vi "Stufen testen.vi"(4 "GD LNI old":bool, 7 "Komponentenauswahl":T5 {"Konzentration" format="%#.6f"}, 8 "error in (no error)":errorcluster caption="Fehler (Eingang, kein Fehler)", 9 "Index Cluster":T4 {"Verdünnungsgas" items=["N2", "O2"]; "Anzahl Stufen" format="%#_5g"}) -> (0 "error out":errorcluster caption="Fehler (Ausgang)", 2 "GD DF":T1)   [LabVIEW 2020, in "Linearisierung v2.lvlib" / "Gasteiler.lvlib"]
uses:
  Gasteiler.lvlib
  KomponentenArray.ctl
  Visualisierungs Elemente/Auswahlfeld.ctl
  Visualisierungs Elemente/Zahlen-Eingabefeld.ctl
  Visualisierungs Elemente/Checkbox(boolsch).ctl
  Aktionen FGV Gasteiler Daten.ctl
  SpanEinstellungen/Aktion FGV GD Errors sammeln.ctl
  SpanEinstellungen/GD Info Cluster.ctl
  LIN ErrorCluster.ctl
  Aktion FGV Gasteilerliste laden.ctl
  AK-Komm Gasteiler/Aktionen AK Komm.ctl
  AK-Komm Gasteiler/Alter Gasteiler/Aktionen AK Komm_ALT.ctl
  Seiten/System Einstellungen V2/Traegergas.ctl
  Horiba/Aktion Befehl.ctl
  Gasteiler Fehler.ctl
  Aktion Lin Daten aufarbeiten.ctl
  Linearisierung v2.lvlib
  Seiten/System Einstellungen V2/System Einstellungen V2.lvlib
  SpanEinstellungen/SpanEinstellungen.lvlib
  AK-Komm Gasteiler/AK Komm Gasteiler.lvlib
  AK-Komm Gasteiler/Alter Gasteiler/Alter Gasteiler.lvlib
  Horiba/Horiba GDC.lvlib
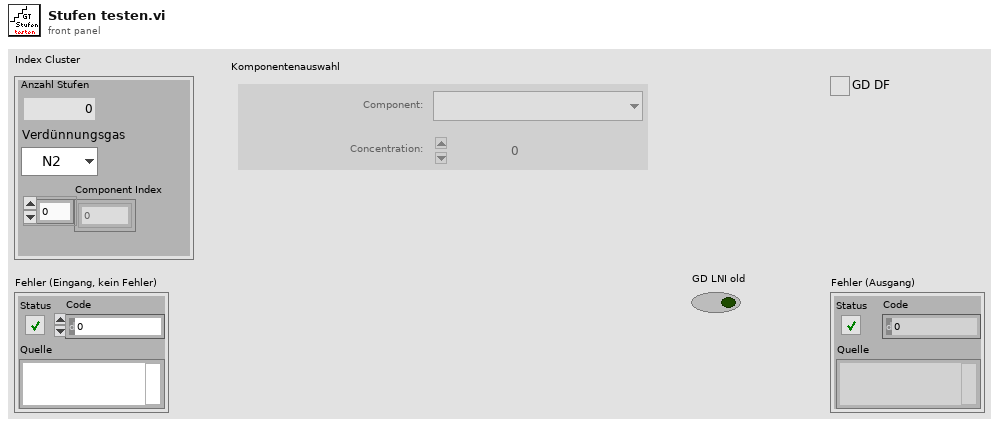
[diagram p1: front panel]
types:
  T1 = typedef "Checkbox(boolsch).ctl" = bool
  T2 = typedef "Zahlen-Eingabefeld.ctl" = sgl
  T3 = typedef "Linearisierung v2.lvlib/Gasteiler.lvlib/Prüfgas in.ctl" = u16
  T4 = cluster{"Anzahl Stufen":T2, "Verdünnungsgas":T3, "Component Index":i32[]}
  T5 = typedef "Linearisierung v2.lvlib/KomponentenArray.ctl" = cluster{"Komponente:":T6, "Konzentration":dbl}[]
  T6 = typedef "Auswahlfeld.ctl" = u16
  T7 = typedef "Linearisierung v2.lvlib/SpanEinstellungen.lvlib/GD Info Cluster.ctl" = cluster{"Wobei":string, "Status":string, "Errors":T8, "Empfangsdaten":string[], "Zeitstempel":string}
  T8 = typedef "Linearisierung v2.lvlib/LIN ErrorCluster.ctl" = cluster{"Störung Kommunikation":bool, "Pressure carrier gas":bool, "Pressure diluted gas":bool, "Outlet Pressure":bool, "SNOX before SAIR":bool, "Störung Gasteiler":bool}
  T9 = typedef "Linearisierung v2.lvlib/SpanEinstellungen.lvlib/Aktion FGV GD Errors sammeln.ctl" = enum16{"lesen", "init", "GD Infos sammeln", "Kalibrierinfos sammeln", "Test Data", "GD Infos selektiv sammeln"}
  T10 = typedef "Linearisierung v2.lvlib/Gasteiler.lvlib/Aktionen FGV Gasteiler Daten.ctl" = enum16{"lesen", "Gasteiler Daten", "Seriellen Param.", "MB-Endwert", "laden", "speichern", "Anforderung", "TCP", "Aufzeichnung Start"}
  T11 = typedef "Linearisierung v2.lvlib/Aktion Lin Daten aufarbeiten.ctl" = enum16{"lesen", "Protkolldaten", "speichern", "laden", "EPA auswerten", "Tabelle schreiben", "Lin auswerten", "Tab init", "Stufentabelle", "EPA aktiviert", "Nachbehandlung laden", "Tabelle löschen", "Istwerte löschen", "Zeile löschen", "Zeile einfügen", "LIN aktiviert", "LIN/EPA aktiv laden", "EGAK Tab", "LIN übernehmen", "Tab init ohne Stufen"}
  T12 = typedef "Linearisierung v2.lvlib/Lin-Polynom Daten.ctl" = cluster{"Messgerät":string, "Kalibrator (Gasteiler)":string, "Bearbeiter/in":string, "Komponente":string, "Zeitstempel":timestamp, "F_max gefordert (%)":sgl, "F_max in %":sgl, "F_max in ppm":sgl, "Vorschlag Ordnung":i32, "Polynom OK":bool, "Polynomkoeff.":dbl[], "Prüfgas Konzentration":dbl, "Pfad EPA":string, "Pfad_LIN":string, "Gasnummer:":u8, "Komponentenauswahl":T5, "Verdünnungsgas":T3, "Zeitdauer Stufe":T2, "Anzahl Stufen":T2, "F_max in % EPA":sgl, "F_max in ppm EPA":sgl, "F_max in % LIN":sgl, "F_max in ppm LIN":sgl, "Punkte umkehren":bool, "EPA Optionsfeld":T13, "Autolin Hovacal":T14, "Spanfactors":sgl[], "Kalibrierauswahl":T15, "Conditions:":T16, "Gasflaschen Nr.:":string, "Bottle Accuracy":dbl, "Konfig Gasflasche":T17, "Gasflasche":T18, "HovaCAL Flow AutoLin":T19, "MFC Output":T20, "Gas Ablaufdatum":timestamp, "Lin Modus":T21, "zusätzliche Zeitdauer Erster Punkt":sgl, "Offsets":sgl[]}
  T13 = typedef "Linearisierung v2.lvlib/EPA Optionsfeld.ctl" = enum32{"Istwert", "Rohwert", "Linearisierter Wert"}
  T14 = typedef "Linearisierung v2.lvlib/Gasteiler.lvlib/HovaCal.lvlib/AutoLin Hovacal.ctl" = enum32{"Keine Auswahl", "Optionsauswahl 1", "Optionsauswahl 2"}
  T15 = typedef "Linearisierung v2.lvlib/Kalibrieroption.ctl" = u16
  T16 = typedef "Linearisierung v2.lvlib/Linearity verification 1065-307.lvlib/Condition.ctl" = u16
  T17 = typedef "System Einstellungen V2.lvlib/Konfig Gasflasche.ctl" = bool
  T18 = typedef "System Einstellungen V2.lvlib/Gasflasche Auswahl.ctl" = u16
  T19 = typedef "Linearisierung v2.lvlib/Gasteiler.lvlib/HovaCAL_Interface.lvlib/Controls.lvlib/Flow Einstellung.ctl" = cluster{"HovaCAL Flow Input Cluster":dbl}
  T20 = typedef "Linearisierung v2.lvlib/Gasteiler.lvlib/HovaCAL_Interface.lvlib/Controls.lvlib/Pump state.ctl" = cluster{"Run":bool}
  T21 = typedef "Linearisierung v2.lvlib/Lin Modus.ctl" = u16
  T22 = typedef "Linearisierung v2.lvlib/Gasteiler.lvlib/Aktion FGV Gasteilerliste laden.ctl" = enum16{"lesen", "laden", "speichern", "Liste erstellen", "Formel ändern", "Gas vereinzeln"}
  T23 = typedef "Linearisierung v2.lvlib/Gasteiler.lvlib/Gasteiler Daten.ctl" = cluster{"Gasteiler":T24, "Gasteiler Stufen":T25, "Gasteiler Type":T26, "Konfig Gasteiler":T27, "Gasteiler Span Eingänge":u16}
  T24 = typedef "String - Eingabefeld.ctl" = string
  T25 = typedef "Linearisierung v2.lvlib/Gasteiler.lvlib/Gasteiler Stufen.ctl" = u16
  T26 = typedef "Linearisierung v2.lvlib/GasteilerType.ctl" = u16
  T27 = typedef "System Einstellungen V2.lvlib/Gasteiler Auswahl.ctl" = u16
  T28 = typedef "Linearisierung v2.lvlib/Gasteiler.lvlib/AK Komm Gasteiler.lvlib/Aktionen AK Komm.ctl" = enum16{"lesen", "initialisieren", "beenden", "Status", "SMAN", "SREM", "STBY", "ASTF", "ASTZ", "SLST", "AGAT", "EGAK", "AGAK", "AKAK", "ADRU", "SKOP", "SVSA", "SVSZ", "SONO", "SAIR", "SNOX", "ANOX", "SSPL", "SRUC", "SLIN", "ALST", "ETYP", "SVIO", "LCYL", "CCYL", "DCYL", "SCYL", "GCYL", "DRGV", "DRDC"}
  T29 = typedef "Linearisierung v2.lvlib/Gasteiler.lvlib/AK Komm Gasteiler.lvlib/Alter Gasteiler.lvlib/Aktionen AK Komm_ALT.ctl" = enum16{"lesen", "initialisieren", "beenden", "SRES", "STBY", "SREM", "SMAN", "SLIN", "SLCH", "SLST", "SSPL", "AGAT", "ALST", "ASTZ", "ASTF", "AGAK", "EGAK"}
  T30 = typedef "System Einstellungen V2.lvlib/Traegergas.ctl" = string
  T31 = typedef "Linearisierung v2.lvlib/Gasteiler.lvlib/Gasteiler Fehler.ctl" = cluster{"Pressure carrier gas":bool, "Pressure diluted gas":bool, "Outlet Pressure":bool, "SNOX before SAIR":bool}
  T32 = typedef "Linearisierung v2.lvlib/Gasteiler.lvlib/Horiba GDC.lvlib/Aktion Befehl.ctl" = enum16{"lesen", "initialisieren", "Beenden", "Standby", "GD/CC", "Info", "Flow", "Alarm", "GD parameter", "GD point", "Durchfluss", "Spuelen1", "Spuelen1 On", "Spuelen1Off", "Spuelen2", "Ventil-Abfrage", "Reset"}
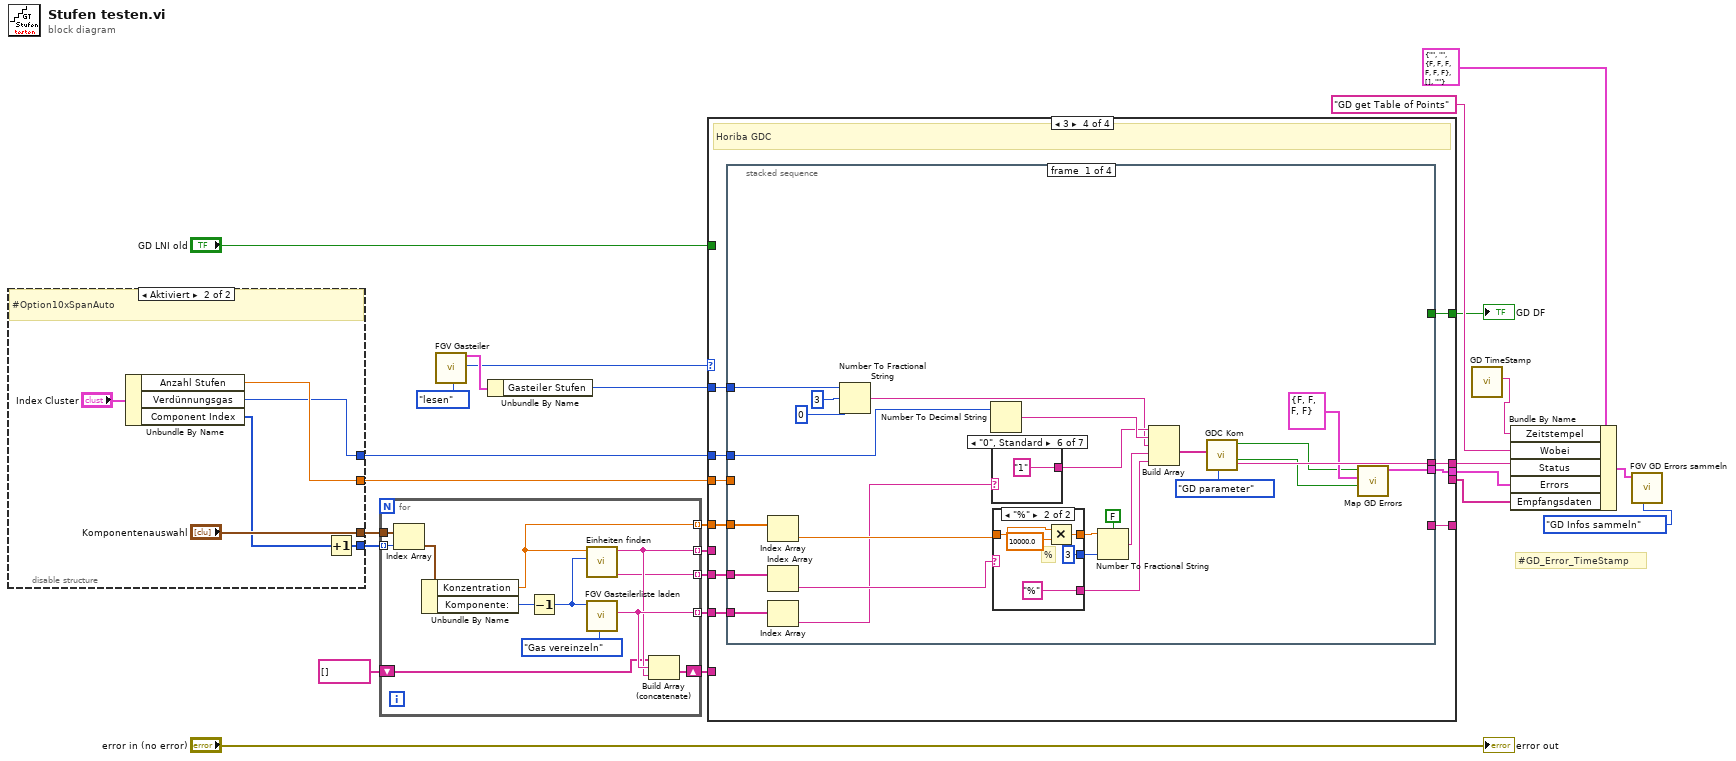
[diagram p0: block diagram]
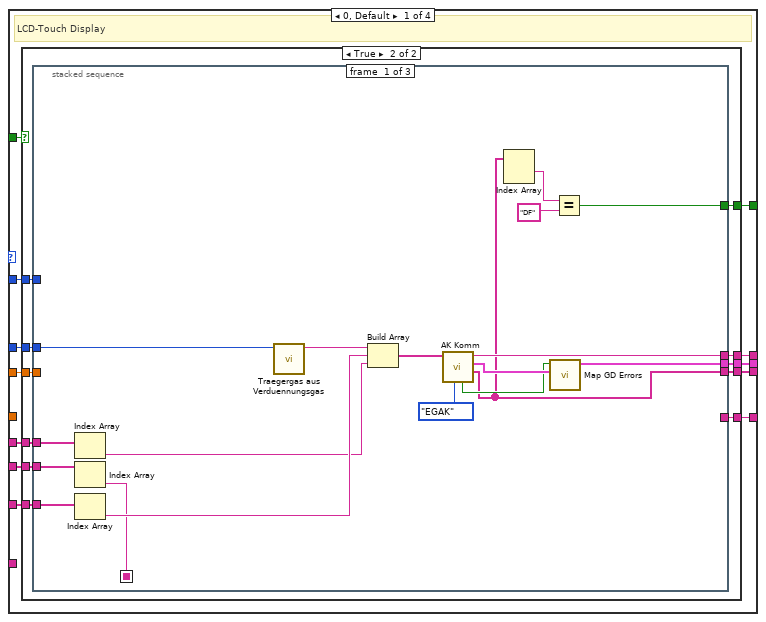
[diagram p2: hidden frame]
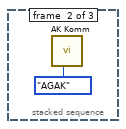
[diagram p4: hidden frame]
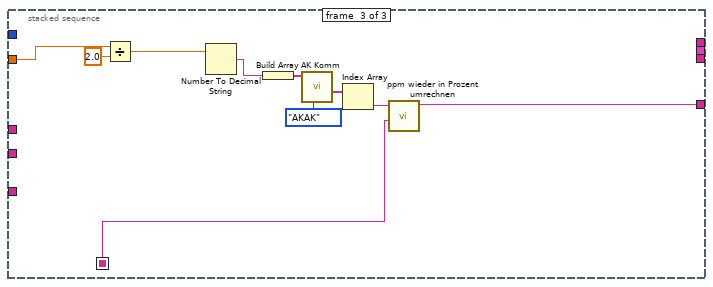
[diagram p5: hidden frame]
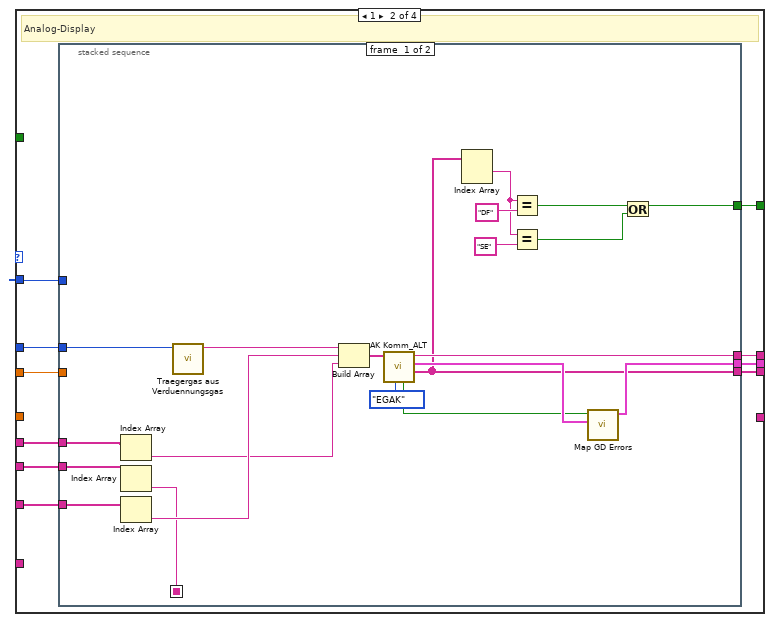
[diagram p6: hidden frame]
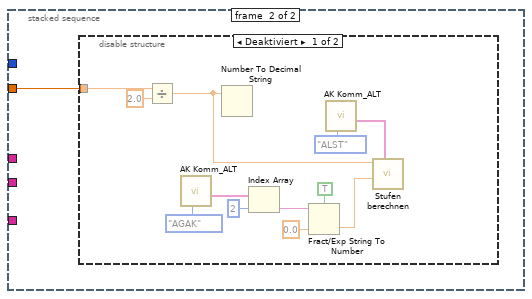
[diagram p7: hidden frame]
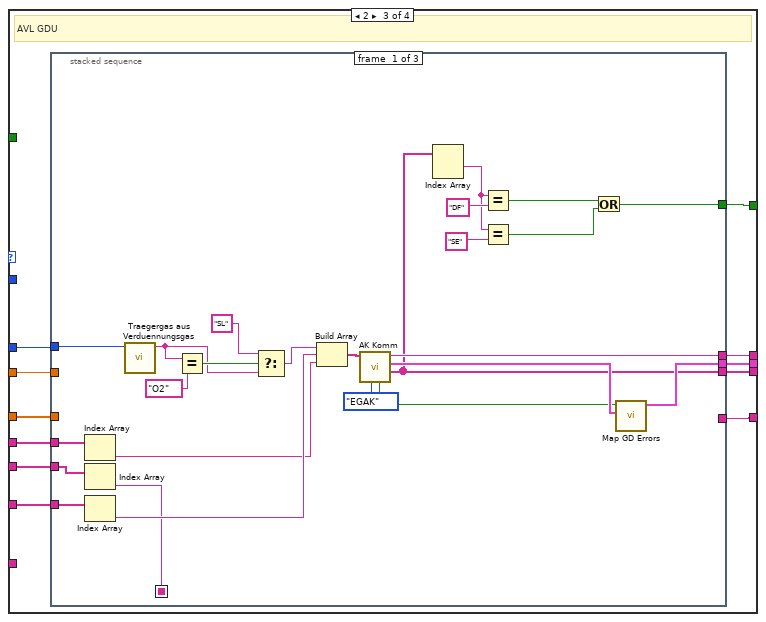
[diagram p9: hidden frame]
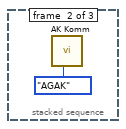
[diagram p10: hidden frame]
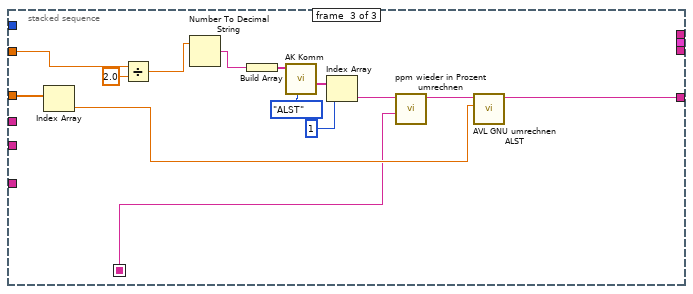
[diagram p11: hidden frame]
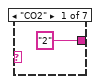
[diagram p12: hidden frame]
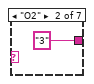
[diagram p13: hidden frame]
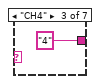
[diagram p14: hidden frame]
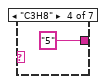
[diagram p15: hidden frame]
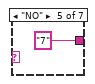
[diagram p16: hidden frame]
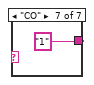
[diagram p17: hidden frame]
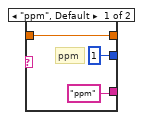
[diagram p18: hidden frame]
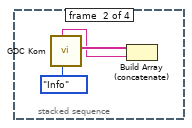
[diagram p19: hidden frame]
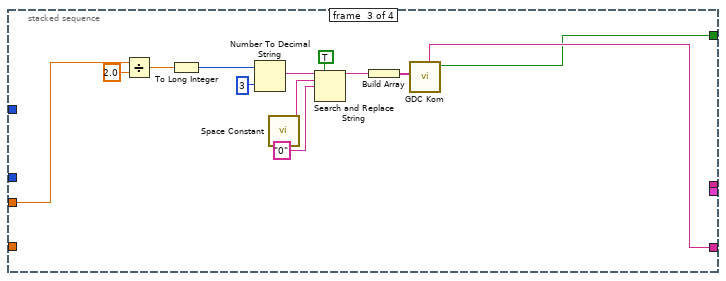
[diagram p20: hidden frame]
diagram:
  # "#GD_Error_TimeStamp"
  n1 = disable-structure shown="Aktiviert" {
    disable-tunnel: [w33 "Komponentenauswahl"] -> w10
    disable-tunnel: [w32 w37] -> w24
    disable-tunnel: [w30 w38] -> w23
    disable-tunnel: [w26 w36] -> w9
    frame Disabled {
      n2 = call "Lin Daten aufarbeiten.vi"("Aktionen"=Aktion_Lin_Daten_aufarbeiten."lesen") -> ("Lin-Polynom"=w31:T12)  [unwired: 16 in, 10 out]
      n3 = call "Lin Daten aufarbeiten.vi"("Aktionen"=Aktion_Lin_Daten_aufarbeiten."lesen") -> ("Lin-Polynom"=w28:T12)  [unwired: 16 in, 10 out]
      n4 = Unbundle By Name(w31) -> ("Komponentenauswahl"=w33:T5, "Gasnummer:"=w26:u8)
      n5 = Unbundle By Name(w31) -> ("Verdünnungsgas"=w32:T3, "Anzahl Stufen"=w30:T2)
      n6 = Unbundle By Name(w28) -> ("Punkte umkehren"=w27:bool)
    }
    frame Enabled {
      # "#Option10xSpanAuto"
      n7 = Unbundle By Name("Index Cluster") -> ("Anzahl Stufen"=w38:T2, "Verdünnungsgas"=w37:T3, "Component Index"=w35:i32[])
      n8 = Increment(x=w35) -> (x+1=w36:i32[])
    }
  }
  n9 = for {
    tunnel: w10 -> [w52]
    tunnel: w9 -> [w51] mode=indexing
    tunnel: [w45] -> w8 mode=indexing
    tunnel: [w46] -> w6 mode=indexing
    shift-right: [w44] -> w5
    shift-left: string[] [] -> [w43]
    tunnel: [w42] -> w7 mode=indexing
    tunnel: [w41] -> w2 mode=indexing
    n10 = Index Array(array=w52, index=w51) -> (element=w49:cluster{"Komponente:":T6, "Konzentration":dbl})
    n11 = Unbundle By Name(w49) -> ("Konzentration"=w41:dbl, "Komponente:"=w48:T6)
    n12 = Decrement(x=w48) -> (x-1=w47:T6)
    n13 = call "Einheiten finden.vi"("Komponente"=w47, "Wert"=w41) -> ("Einheit in String"=w42:string, "String"=w45:string)  [unwired: 5 in, 3 out]
    n14 = call "FGV Gasteilerliste laden.vi"("Aktion"=Aktion_FGV_Gasteilerliste_laden."Gas vereinzeln", "Gasindex"=w47) -> ("Formel"=w46:string)  [unwired: 7 in, 2 out]
    n15 = Build Array (concatenate)(w43, w46, w45) -> (w44:string[])
  }
  n16 = call "FGV Gasteiler.vi"("Aktionen"=Aktionen_FGV_Gasteiler_Daten."lesen") -> ("Gasteiler Daten"=w22:T23, "Gasteiler Type"=w20:T26)  [unwired: 11 in, 6 out]
  n17 = Unbundle By Name(w22) -> ("Gasteiler Stufen"=w19:T25)
  n18 = case shown="3" w20 {
    tunnel: w19 -> [w64 w114 _ w209]
    tunnel: w24 -> [w63 w112 w155 w207]
    tunnel: w23 -> [w62 w113 w159 w208]
    tunnel: [w61 w111 w158 w206] -> w15
    tunnel: [w59 w109 w156 w205] -> w14
    tunnel: [w60 w110 w157 _] -> w13
    tunnel: w8 -> [w56 w107 w154 _]
    tunnel: w7 -> [w55 w106 w153 w203]
    tunnel: w6 -> [w58 w108 w152 w200]
    tunnel: w5 -> [_ _ _ _]
    tunnel: "GD LNI old" -> [w57 _ _ _]
    tunnel: [w54 _ w149 w202] -> _
    tunnel: [w53 w105 w151 w201] -> w3
    tunnel: w2 -> [_ _ w150 w204]
    frame 0, Default {
      # "LCD-Touch Display"
      n19 = case shown="True" w57 {
        tunnel: w64 -> [_ w75]
        tunnel: w63 -> [_ w74]
        tunnel: w62 -> [_ w73]
        tunnel: [_ w72] -> w61
        tunnel: [_ w71] -> w60
        tunnel: [_ w70] -> w59
        tunnel: w58 -> [_ w69]
        tunnel: w56 -> [_ w68]
        tunnel: w55 -> [_ w67]
        tunnel: [_ w66] -> w54
        tunnel: [_ w65] -> w53
        frame False {
        }
        frame True {
          n20 = stacked-sequence {
            seq-local: [w80 _ _] -> [_ _ w103]
            tunnel: w75 -> [_ _ _]
            tunnel: w74 -> [w92 _ _]
            tunnel: w73 -> [_ _ w101]
            tunnel: [w89 _ _] -> w72
            tunnel: [w79 _ _] -> w71
            tunnel: [w87 _ _] -> w70
            tunnel: w69 -> [w85 _ _]
            tunnel: w68 -> [w83 _ _]
            tunnel: w67 -> [w81 _ _]
            tunnel: [_ _ w95] -> w66
            tunnel: [w76 _ _] -> w65
            frame #0 {
              n21 = Index Array(array=w83) -> (element=w82:string)  [unwired: 1 in]
              n22 = Index Array(array=w81) -> (element=w80:string)  [unwired: 1 in]
              n23 = Index Array(array=w85) -> (element=w84:string)  [unwired: 1 in]
              n24 = call "Traegergas aus Verduennungsgas.vi"("Verdünnungsgas"=w92) -> ("Trägergas"=w91:T30)  [unwired: 10 in]
              n25 = Build Array(w91, w84, w82) -> (w90:T30[])
              n26 = call "AK Komm.vi"("Aktionen"=Aktionen_AK_Komm."EGAK", "Daten"=w90) -> ("Empfangsdaten"=w79:string[], "Error"=w88:T31, "Status"=w89:string, "Störung Kommunikation"=w86:bool)  [unwired: 3 in, 3 out]
              n27 = Index Array(array=w79) -> (element #1=w77:string)  [unwired: 2 in, 1 out]
              n28 = call "Map GD Errors.vi"("Error"=w88, "Störung Kommunikation"=w86) -> ("LIN Errors-Cluster (Ausgang)"=w87:T8)  [unwired: 8 in, 1 out]
              n29 = Equal?(x=w77, y="DF") -> (x = y?=w76:bool)
            }
            frame #1 {
              n30 = call "AK Komm.vi"("Aktionen"=Aktionen_AK_Komm."AGAK") -> ()  [unwired: 4 in, 7 out]
            }
            frame #2 {
              n31 = Divide(x=w101, y=T2 2.0) -> (x/y=w100:T2)
              n32 = Number To Decimal String(number=w100) -> (decimal integer string=w104:string)  [unwired: 1 in]
              n33 = Build Array(w104) -> (w98:string[])
              n34 = call "AK Komm.vi"("Aktionen"=Aktionen_AK_Komm."AKAK", "Daten"=w98) -> ("Empfangsdaten"=w97:string[])  [unwired: 3 in, 6 out]
              n35 = Index Array(array=w97) -> (element=w96:string)  [unwired: 1 in]
              n36 = call "ppm wieder in Prozent umrechnen.vi"("Einheit"=w103, "Werteingang"=w96) -> ("Wertausgang"=w95:string)  [unwired: 9 in]
            }
          }
        }
      }
    }
    frame 1 {
      # "Analog-Display"
      n37 = stacked-sequence {
        seq-local: [w122 _] -> [_ _]
        tunnel: w114 -> [_ _]
        tunnel: w113 -> [_ w136]
        tunnel: w112 -> [w134 _]
        tunnel: [w131 _] -> w111
        tunnel: [w129 _] -> w109
        tunnel: [w120 _] -> w110
        tunnel: w108 -> [w127 _]
        tunnel: w107 -> [w125 _]
        tunnel: w106 -> [w123 _]
        tunnel: [w116 _] -> w105
        frame #0 {
          n38 = Index Array(array=w125) -> (element=w124:string)  [unwired: 1 in]
          n39 = Index Array(array=w123) -> (element=w122:string)  [unwired: 1 in]
          n40 = Index Array(array=w127) -> (element=w126:string)  [unwired: 1 in]
          n41 = call "Traegergas aus Verduennungsgas.vi"("Verdünnungsgas"=w134) -> ("Trägergas"=w133:T30)  [unwired: 10 in]
          n42 = Build Array(w133, w126, w124) -> (w132:T30[])
          n43 = call "AK Komm_ALT.vi"("Aktionen_ALT"=Aktionen_AK_Komm_ALT."EGAK", "Daten"=w132) -> ("Empfangsdaten"=w120:string[], "Error"=w130:T31, "Status"=w131:string, "Störung Kommunikation"=w128:bool)  [unwired: 5 in, 1 out]
          n44 = Index Array(array=w120) -> (element #1=w118:string)  [unwired: 2 in, 1 out]
          n45 = Equal?(x=w118, y="DF") -> (x = y?=w119:bool)
          n46 = Equal?(x=w118, y="SE") -> (x = y?=w115:bool)
          n47 = call "Map GD Errors.vi"("Error"=w130, "Störung Kommunikation"=w128) -> ("LIN Errors-Cluster (Ausgang)"=w129:T8)  [unwired: 8 in, 1 out]
          n48 = Or(x=w119, y=w115) -> (x .or. y?=w116:bool)
        }
        frame #1 {
          n49 = disable-structure shown="Deaktiviert" {
            disable-tunnel: w136 -> [w138 _]
            frame Disabled {
              n50 = Divide(x=w138, y=T2 2.0) -> (x/y=w137:T2)
              n51 = call "AK Komm_ALT.vi"("Aktionen_ALT"=Aktionen_AK_Komm_ALT."AGAK") -> ("Empfangsdaten"=w145:string[])  [unwired: 6 in, 4 out]
              n52 = Number To Decimal String(number=w137) -> ()  [unwired: 1 in, 1 out]
              n53 = Index Array(array=w145, index=2 ("Index")) -> (element=w142:string)
              n54 = Fract/Exp String To Number(use system decimal point (T)=TRUE ("Systemdezimalzeichen verwenden (T)"), string=w142, default (0 dbl)=sgl 0.0 ("Standard (0 DBL)")) -> (number=w141:sgl)  [unwired: 1 in, 1 out]
              n55 = call "AK Komm_ALT.vi"("Aktionen_ALT"=Aktionen_AK_Komm_ALT."ALST") -> ("Empfangsdaten"=w147:string[])  [unwired: 6 in, 4 out]
              n56 = call "Stufen berechnen.vi"("Empfangsdaten"=w147, "Konzentration"=w141, "Stufen"=w137) -> ()  [unwired: 7 in, 2 out]
            }
            frame Enabled {
            }
          }
        }
      }
    }
    frame 2 {
      # "AVL GDU"
      n57 = stacked-sequence {
        seq-local: [w167 _ _] -> [_ _ w187]
        tunnel: w155 -> [w183 _ _]
        tunnel: w159 -> [_ _ w197]
        tunnel: [w176 _ _] -> w158
        tunnel: [w161 _ _] -> w157
        tunnel: [w173 _ _] -> w156
        tunnel: w154 -> [w172 _ _]
        tunnel: w153 -> [w171 _ _]
        tunnel: w152 -> [w170 _ _]
        tunnel: [w160 _ _] -> w151
        tunnel: w150 -> [_ _ w195]
        tunnel: [_ _ w189] -> w149
        frame #0 {
          n58 = Index Array(array=w172) -> (element=w168:string)  [unwired: 1 in]
          n59 = Index Array(array=w171) -> (element=w167:string)  [unwired: 1 in]
          n60 = Index Array(array=w170) -> (element=w169:string)  [unwired: 1 in]
          n61 = call "Traegergas aus Verduennungsgas.vi"("Verdünnungsgas"=w183) -> ("Trägergas"=w179:T30)  [unwired: 10 in]
          n62 = Equal?(x=w179, y=T30 "O2") -> (x = y?=w181:bool)
          n63 = Select(t="SL" ("Formel"), s=w181, f=w179) -> (s? t:f=w178:T30)
          n64 = Build Array(w178, w169, w168) -> (w177:T30[])
          n65 = call "AK Komm.vi"("Aktionen"=Aktionen_AK_Komm."EGAK", "Daten"=w177) -> ("Empfangsdaten"=w161:string[], "Error"=w175:T31, "Status"=w176:string, "Störung Kommunikation"=w174:bool)  [unwired: 3 in, 3 out]
          n66 = Index Array(array=w161) -> (element #1=w164:string)  [unwired: 2 in, 1 out]
          n67 = Equal?(x=w164, y="DF") -> (x = y?=w165:bool)
          n68 = Equal?(x=w164, y="SE") -> (x = y?=w162:bool)
          n69 = Or(x=w165, y=w162) -> (x .or. y?=w160:bool)
          n70 = call "Map GD Errors.vi"("Error"=w175, "Störung Kommunikation"=w174) -> ("LIN Errors-Cluster (Ausgang)"=w173:T8)  [unwired: 8 in, 1 out]
        }
        frame #1 {
          n71 = call "AK Komm.vi"("Aktionen"=Aktionen_AK_Komm."AGAK") -> ()  [unwired: 4 in, 7 out]
        }
        frame #2 {
          n72 = Index Array(array=w195) -> (element=w194:dbl)  [unwired: 1 in]
          n73 = Divide(x=w197, y=T2 2.0) -> (x/y=w196:T2)
          n74 = Number To Decimal String(number=w196) -> (decimal integer string=w199:string)  [unwired: 1 in]
          n75 = Build Array(w199) -> (w192:string[])
          n76 = call "AK Komm.vi"("Aktionen"=Aktionen_AK_Komm."ALST", "Daten"=w192) -> ("Empfangsdaten"=w191:string[])  [unwired: 3 in, 6 out]
          n77 = Index Array(array=w191, index=1 ("Index")) -> (element=w188:string)
          n78 = call "ppm wieder in Prozent umrechnen.vi"("Einheit"=w187, "Werteingang"=w188) -> ("Wertausgang"=w186:string)  [unwired: 9 in]
          n79 = call "AVL GNU umrechnen ALST.vi"("Konzentration"=w194, "Teilerstufe in%"=w186) -> ("Konzentration"=w189:string)  [unwired: 9 in]
        }
      }
    }
    frame 3 {
      # "Horiba GDC"
      n80 = stacked-sequence {
        tunnel: w209 -> [w222 _ _ _]
        tunnel: w208 -> [_ _ w264 _]
        tunnel: w207 -> [w221 _ _ _]
        tunnel: [w220 _ _ _] -> w206
        tunnel: [w219 _ _ _] -> w205
        tunnel: w204 -> [w215 _ _ _]
        tunnel: w203 -> [w213 _ _ _]
        tunnel: [_ _ w256 _] -> w202
        tunnel: [_ _ w255 _] -> w201
        tunnel: w200 -> [w211 _ _ _]
        frame #0 {
          n81 = Index Array(array=w215) -> (element=w214:dbl)  [unwired: 1 in]
          n82 = Index Array(array=w213) -> (element=w212:string)  [unwired: 1 in]
          n83 = Index Array(array=w211) -> (element=w210:string)  [unwired: 1 in]
          n84 = Number To Fractional String(number=w222, width (-)=i16 3 ("Breite (-)"), precision (6)=i16 0 ("Genauigkeit (6)")) -> (F-format string=w223:string)  [unwired: 1 in]
          n85 = Number To Decimal String(number=w221) -> (decimal integer string=w229:string)  [unwired: 1 in]
          n86 = case shown="\"0\", Standard" w210 {
            tunnel: ["2" "3" "4" "5" "7" "1" "1"] -> w224
            frame "CO2" {
            }
            frame "O2" {
            }
            frame "CH4" {
            }
            frame "C3H8" {
            }
            frame "NO" {
            }
            frame "0", Default {
            }
            frame "CO" {
            }
          }
          n87 = case shown="\"%\"" w212 {
            tunnel: [i16 1 ("Genauigkeit (6)") i16 3 ("Genauigkeit (6)")] -> w233
            tunnel: w214 -> [w243 w248]
            tunnel: [w243 w247] -> w234
            tunnel: ["ppm" "%"] -> w231
            frame "ppm", Default {
              # "ppm"
            }
            frame "%" {
              # "%"
              n88 = Multiply(x=w248, y=T2 10000.0) -> (x*y=w247:dbl)
            }
          }
          n89 = Number To Fractional String(use system decimal point (T)=FALSE ("Systemdezimalzeichen verwenden (T)"), number=w234, precision (6)=w233) -> (F-format string=w230:string)  [unwired: 1 in]
          n90 = Build Array(w224, w229, w223, w230, w231) -> (w227:string[])
          n91 = call "GDC Kom.vi"("Befehl"=Aktion_Befehl."GD parameter", "Daten"=w227) -> ("Status (alarm)"=w216:bool, "Fehler"=w217:bool, "Status"=w220:string)  [unwired: 3 in, 4 out]
          n92 = call "Map GD Errors.vi"("Störung Gasteiler"=w216, "Error"=T31 {"Pressure carrier gas"=FALSE, "Pressure diluted gas"=FALSE, "Outlet Pressure"=FALSE, "SNOX before SAIR"=FALSE}, "Störung Kommunikation"=w217) -> ("LIN Errors-Cluster (Ausgang)"=w219:T8)  [unwired: 7 in, 1 out]
        }
        frame #1 {
          n93 = call "GDC Kom.vi"("Befehl"=Aktion_Befehl."Info") -> ("Gas"=w251:string[], "Konzentration 2"=w250:string)  [unwired: 4 in, 5 out]
          n94 = Build Array (concatenate)(w251, w250) -> ()  [unwired: 1 out]
        }
        frame #2 {
          n95 = Divide(x=w264, y=T2 2.0) -> (x/y=w260:T2)
          n96 = To Long Integer(number=w260) -> (32bit integer=w259:i32)
          n97 = Number To Decimal String(number=w259, width (-)=i16 3 ("Breite (-)")) -> (decimal integer string=w262:string)
          n98 = call <vilib>:"Space Constant.vi"() -> ("String"=w254:string)
          n99 = Search and Replace String(replace all?=TRUE ("Alle ersetzen? (F)"), input string=w262, search string=w254, replace string="0" ("Ersetzungs-String (\"\")")) -> (result string=w257:string)  [unwired: 4 in, 3 out]
          n100 = Build Array(w257) -> (w258:string[])
          n101 = call "GDC Kom.vi"("Daten"=w258) -> ("Fehler"=w255:bool, "Konzentration"=w256:string)  [unwired: 4 in, 5 out]
        }
        frame #3 {
          n102 = call "GDC Kom.vi"("Befehl"=Aktion_Befehl."Standby") -> ()  [unwired: 4 in, 7 out]
        }
      }
    }
  }
  "GD DF" <- w3
  n103 = call "GD TimeStamp.vi"() -> ("date/time string"=w1:string)  [unwired: 10 in, 1 out]
  n104 = Bundle By Name(cluster=T7 {"Wobei"="", "Status"="", "Errors"={"Störung Kommunikation"=FALSE, "Pressure carrier gas"=FALSE, "Pressure diluted gas"=FALSE, "Outlet Pressure"=FALSE, "SNOX before SAIR"=FALSE, "Störung Gasteiler"=FALSE}, "Empfangsdaten"=[], "Zeitstempel"=""} ("GD Info-Cluster"), "Zeitstempel"=w1, "Wobei"="GD get Table of Points" ("Status"), "Status"=w15, "Errors"=w14, "Empfangsdaten"=w13) -> (w12:T7)
  n105 = call "FGV GD Errors sammeln.vi"("Aktion"=Aktion_FGV_GD_Errors_sammeln."GD Infos sammeln", "GD Info-Cluster in"=w12) -> ()  [unwired: 7 in, 3 out]
  "error out" <- "error in (no error)"
